vi "Teleop.vi"(10 "Match Info":T1={"Autonomous Elapsed Seconds"=0.0, "TeleOp Elapsed Seconds"=0.0, "Disabled Elapsed Seconds"=0.0, "Visited Autonomous"=FALSE, "Visited TeleOp"=FALSE, "Visited Disabled"=FALSE, "Autonomous Settings"={"Autonomous Style"=enum."Independent", "VI Refnum"=refnum}}, 11 "Call Context":T2) -> ()   [LabVIEW 2012]
doc: "This VI is called for each TeleOp packet received from the DS where the robot is not disabled. It is often used to read from the joysticks and update I/O or to update setpoints for timed control loops. It should complete and return within 20 milliseconds or it may miss DS packets."
uses:
  <vilib>/Rock Robotics/WPI/DriverStation/WPI_DriverStationDerivedRobotMode.ctl
  <vilib>/Rock Robotics/WPI/DriverStation/WPI_DriverStationMatch Info.ctl
  <vilib>/Rock Robotics/WPI/Relay/WPI_RelayValue.ctl
  Robot Global Data.vi
  <vilib>/Rock Robotics/WPI/Joystick/WPI_JoystickGetSetRefNum.vi
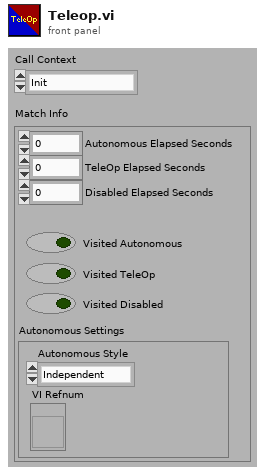
[diagram p1: front panel]
types:
  T1 = typedef "WPI_DriverStationMatch Info.ctl" = cluster{"Autonomous Elapsed Seconds":dbl, "TeleOp Elapsed Seconds":dbl, "Disabled Elapsed Seconds":dbl, "Visited Autonomous":bool, "Visited TeleOp":bool, "Visited Disabled":bool, "Autonomous Settings":cluster{"Autonomous Style":enum16{"Iterative", "Independent"}, "VI Refnum":refnum<vi>}}
  T2 = typedef "WPI_DriverStationDerivedRobotMode.ctl" = enum16{"Init", "Execute", "Stop"}
  T3 = typedef "WPI_RelayValue.ctl" = enum16{"Off", "On", "Forward", "Reverse"}
  T4 = typedef "WPI_JoystickDevRef.ctl" = cluster{"Device":T5}
  T5 = typedef "WPI_JoystickDeviceEnum.ctl" = enum16{"USB 1", "USB 2", "USB 3", "USB 4", "Kinect 1", "Kinect 2"}
  T6 = cluster{"axis 1 (x)":dbl, "axis 2 (y)":dbl, "axis 3 (throttle)":dbl, "axis 4":dbl, "axis 5":dbl, "axis 6":dbl}
  T7 = typedef "WPI_RelayDevRef.ctl" = cluster{"DevStatus":errorcluster, "Relay Channel":T8, "Digital Module":T9, "Relay Direction":T10}
  T8 = typedef "FPGA_DIORelayChannel.ctl" = enum8{"Relay 1", "Relay 2", "Relay 3", "Relay 4", "Relay 5", "Relay 6", "Relay 7", "Relay 8", "Invalid"}
  T9 = typedef "FPGA_TypedefDigitalModule.ctl" = enum16{"Digital Module 1", "Digital Module 2"}
  T10 = typedef "WPI_RelayDirection.ctl" = enum16{"Both directions", "Forward only", "Reverse only"}
  T11 = cluster{"Driver Station Digital Input (1-8)[0]":bool, "Driver Station Digital Input (1-8)[1]":bool, "Driver Station Digital Input (1-8)[2]":bool, "Driver Station Digital Input (1-8)[3]":bool, "Driver Station Digital Input (1-8)[4]":bool, "Driver Station Digital Input (1-8)[5]":bool, "Driver Station Digital Input (1-8)[6]":bool, "Driver Station Digital Input (1-8)[7]":bool, "Driver Station Digital Input (1-8)[8]":bool}
  T12 = cluster{"Shifting":cluster{"Right Servo High":dbl, "Right Servo Low":dbl, "Left Servo High":dbl, "Left Servo Low":dbl}, "Breaking":cluster{"Coast Position":dbl, "Break Position":dbl}}
  T13 = typedef "WPI_JoystickButtonState.ctl" = cluster{"Button 1":bool, "Button 2":bool, "Button 3":bool, "Button 4":bool, "Button 5":bool, "Button 6":bool, "Button 7":bool, "Button 8":bool, "Button 9":bool, "Button 10":bool, "Button 11":bool, "Button 12":bool}
  T14 = typedef "WPI_MotorControlDeviceRef.ctl" = cluster{"DeviceStatus":errorcluster, "Type":enum16{"PWM", "CAN"}, "PWM":cluster{"Digital Module":T9, "PWM Channel":T15, "DeadBand":T16}, "CAN":cluster{"Device Number":u8, "Control Mode":T17, "Semaphore":T18, "Max Vout":dbl}, "Invert":bool, "TransformRef":T19, "InvTransformRef":T19}
  T15 = typedef "FPGA_DIOPWMChannel.ctl" = enum8{"PWM 1", "PWM 2", "PWM 3", "PWM 4", "PWM 5", "PWM 6", "PWM 7", "PWM 8", "PWM 9", "PWM 10", "Invalid"}
  T16 = typedef "WPI_PWMDeadband.ctl" = cluster{"Name":string, "maxPositivePwm":i32, "minPositivePwm":i32, "centerPwm":i32, "maxNegativePwm":i32, "minNegativePwm":i32, "angularRange":u16}
  T17 = typedef "WPI_CANJaguar_ControlMode.ctl" = enum8{"Percent VBus", "Current", "Speed", "Position", "Voltage"}
  T18 = typedef "Semaphore RefNum" = refnum<k1>
  T19 = typedef "WPI_PWMTransform_ConPane.ctl" = refnum<vi>
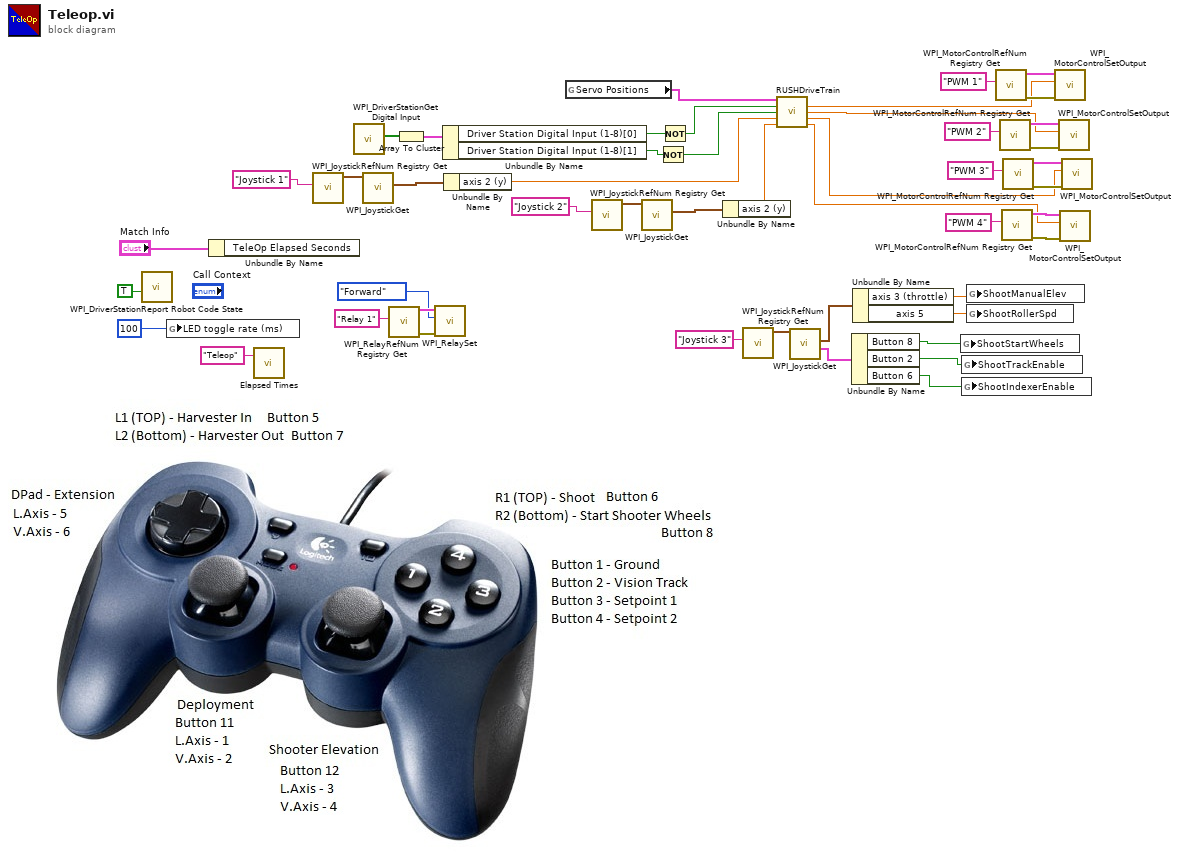
[diagram p0: block diagram]
diagram:
  n1 = call <vilib>:"WPI_DriverStationReport Robot Code State.vi"("TeleOp"=TRUE ("Autonomous")) -> ()  [unwired: 10 in, 1 out]
  n2 = global write "Robot Global Data.vi" "LED toggle rate (ms)"(u32 100 ("LED ms toggle rate")) -> ()
  n3 = Unbundle By Name("Match Info") -> ()  [unwired: 1 out]
  n4 = call "Elapsed Times.vi"("Call Name"="Teleop") -> ()  [unwired: 2 in, 1 out]
  n5 = call <vilib>:"WPI_JoystickRefNum Registry Get.vi"("refnum name"="Joystick 1") -> ("JoystickDevRef"=w31:T4)  [unwired: 1 in, 9 out]
  n6 = call <vilib>:"WPI_DriverStationGet Digital Input.vi"() -> ("Driver Station Digital Input (1-8)"=w26:bool[])  [unwired: 11 in]
  n7 = call <vilib>:"WPI_JoystickGet.vi"("JoystickDevRef"=w31) -> ("Axes"=w30:T6)  [unwired: 1 in, 5 out]
  n8 = call <vilib>:"WPI_RelayRefNum Registry Get.vi"("refnum name"="Relay 1") -> ("error out"=w42:errorcluster, "RelayDevRef"=w44:T7)  [unwired: 9 in]
  n9 = Array To Cluster(array=w26) -> (cluster=w25:T11)
  n10 = call <vilib>:"WPI_RelaySet.vi"("error in (no error)"=w42, "RelayValue"=WPI_RelayValue."Forward", "RelayDevRef"=w44) -> ()  [unwired: 7 in, 2 out]
  n11 = Unbundle By Name(w25) -> ("Driver Station Digital Input (1-8)[0]"=w24:bool, "Driver Station Digital Input (1-8)[1]"=w23:bool)
  n12 = Unbundle By Name(w30) -> ("axis 2 (y)"=w20:dbl)
  n13 = global read "Robot Global Data.vi" "Servo Positions"() -> (w18:T12)
  n14 = call <vilib>:"WPI_JoystickRefNum Registry Get.vi"("refnum name"="Joystick 2") -> ("JoystickDevRef"=w28:T4)  [unwired: 1 in, 9 out]
  n15 = call <vilib>:"WPI_JoystickGet.vi"("JoystickDevRef"=w28) -> ("Axes"=w29:T6)  [unwired: 1 in, 5 out]
  n16 = Not(x=w23) -> (.not. x?=w21:bool)
  n17 = Not(x=w24) -> (.not. x?=w22:bool)
  n18 = Unbundle By Name(w29) -> ("axis 2 (y)"=w19:dbl)
  n19 = call <vilib>:"WPI_JoystickRefNum Registry Get.vi"("refnum name"="Joystick 3") -> ("JoystickDevRef"=w40:T4)  [unwired: 9 in, 1 out]
  n20 = call "RUSHDriveTrain.vi"("Servo Positions"=w18, "Low Gear + Brake"=w22, "Low Gear"=w21, "LeftJoystick"=w20, "RightJoystick"=w19) -> ("Left Drive"=w5:dbl, "Right Drive"=w4:dbl, "Left Servo"=w3:dbl, "Right Servo"=w2:dbl)  [unwired: 6 in, 1 out]
  n21 = call <vilib>:"WPI_JoystickGet.vi"("JoystickDevRef"=w40) -> ("Buttons"=w38:T13, "Axes"=w37:T6)  [unwired: 4 in, 1 out]
  n22 = Unbundle By Name(w38) -> ("Button 8"=w34:bool, "Button 2"=w35:bool, "Button 6"=w36:bool)
  n23 = Unbundle By Name(w37) -> ("axis 3 (throttle)"=w33:dbl, "axis 5"=w1:dbl)
  n24 = global write "Robot Global Data.vi" "ShootStartWheels"(w34) -> ()
  n25 = global write "Robot Global Data.vi" "ShootTrackEnable"(w35) -> ()
  n26 = global write "Robot Global Data.vi" "ShootIndexerEnable"(w36) -> ()
  n27 = global write "Robot Global Data.vi" "ShootManualElev"(w33) -> ()
  n28 = global write "Robot Global Data.vi" "ShootRollerSpd"(w1) -> ()
  n29 = call <vilib>:"WPI_MotorControlRefNum Registry Get.vi"("refnum name"="PWM 1") -> ("error out"=w6:errorcluster, "MotorControlDevRef"=w7:T14)  [unwired: 9 in]
  n30 = call <vilib>:"WPI_MotorControlRefNum Registry Get.vi"("refnum name"="PWM 2") -> ("error out"=w11:errorcluster, "MotorControlDevRef"=w10:T14)  [unwired: 9 in]
  n31 = call <vilib>:"WPI_MotorControlRefNum Registry Get.vi"("refnum name"="PWM 4") -> ("error out"=w17:errorcluster, "MotorControlDevRef"=w16:T14)  [unwired: 9 in]
  n32 = call <vilib>:"WPI_MotorControlRefNum Registry Get.vi"("refnum name"="PWM 3") -> ("error out"=w12:errorcluster, "MotorControlDevRef"=w13:T14)  [unwired: 9 in]
  n33 = call <vilib>:"WPI_MotorControlSetOutput.vi"("error in (no error)"=w6, "Output"=w5, "MotorControlDevRef"=w7) -> ()  [unwired: 6 in, 3 out]
  n34 = call <vilib>:"WPI_MotorControlSetOutput.vi"("error in (no error)"=w11, "Output"=w4, "MotorControlDevRef"=w10) -> ()  [unwired: 6 in, 3 out]
  n35 = call <vilib>:"WPI_MotorControlSetOutput.vi"("error in (no error)"=w17, "Output"=w2, "MotorControlDevRef"=w16) -> ()  [unwired: 6 in, 3 out]
  n36 = call <vilib>:"WPI_MotorControlSetOutput.vi"("error in (no error)"=w12, "Output"=w3, "MotorControlDevRef"=w13) -> ()  [unwired: 6 in, 3 out]
